vi "AlliGator Read HDF5 FLI Image Information.vi"(8 "error in (no error)":errorcluster, 11 "ref in":T3 format="%.0x") -> (0 "error out":errorcluster, 1 "Image Information":string, 2 "Image Binning Options":T1={"Use Image Binning"=FALSE, "X Bin"=1, "Y Bin"=1} {"Y Bin" min=1; "X Bin" min=1}, 3 "Image ROI Information":T2)   [LabVIEW 2021, in "AlliGator HDF5.lvlib"]
doc: "Reads HDF5 FLI dataset image information."
uses:
  AlliGator HDF5.lvlib
  <vilib>/addons/h5labview2/base/hid_t.ctl
  SwissSPAD/SwissSPAD Live_Image ROI Information.ctl
  AlliGator Image Binning Options.ctl
  <vilib>/addons/h5labview2/base/lib_path.vi
  <vilib>/addons/h5labview2/base/H5Equery.vi
  <vilib>/addons/h5labview2/dataset/H5Dread.llb/H5Dread.xnode
  SwissSPAD/SwissSPAD Live.lvlib
  AlliGator Source Image.lvlib
  <vilib>/addons/h5labview2/group/H5G.lvlib
  Variant/Variant.lvlib
panel:
  # "see the AlliGator License on the block diagram (Ctrl+E or Window:Show Block Diagram)"
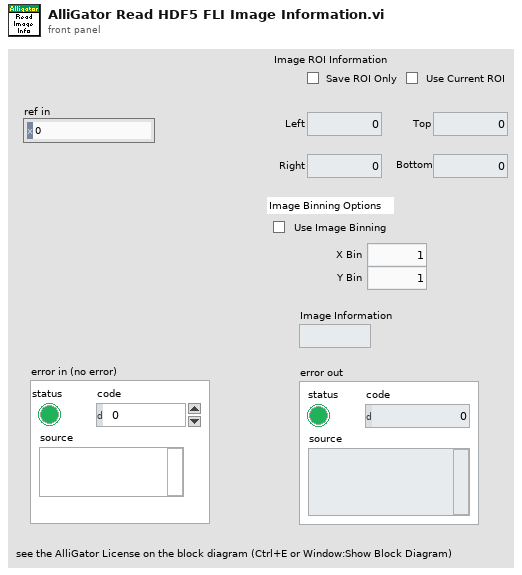
[diagram p1: front panel]
types:
  T1 = typedef "AlliGator Source Image.lvlib/AlliGator Image Binning Options.ctl" = cluster{"Use Image Binning":bool, "X Bin":i32, "Y Bin":i32}
  T2 = typedef "SwissSPAD Live.lvlib/SwissSPAD Live_Image ROI Information.ctl" = cluster{"Save ROI Only":bool, "Left":u16, "Top":u16, "Right":u16, "Bottom":u16, "Use Current ROI":bool}
  T3 = typedef "hid_t.ctl" = i64
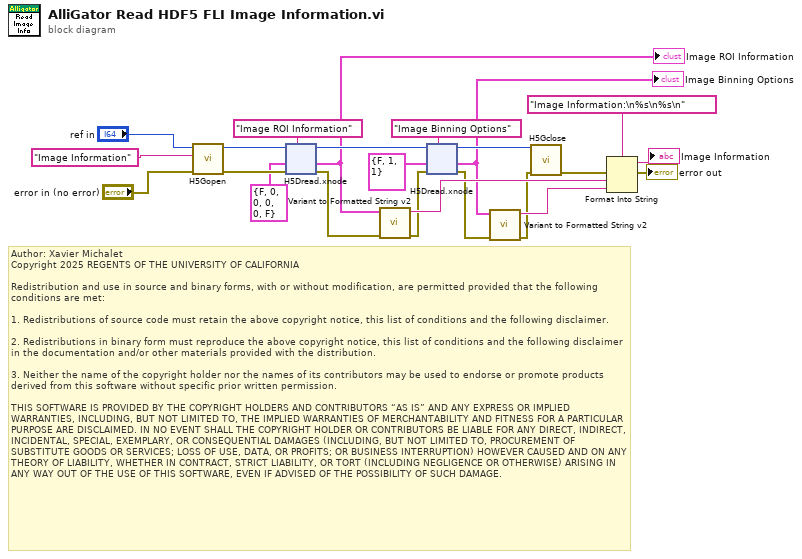
[diagram p0: block diagram]
diagram:
  # "Author: Xavier Michalet\nCopyright 2025 REGENTS OF THE UNIVERSITY OF CALIFORNIA\n\nRedistribution and use in source and binary forms, with or without modification, are permitted provided that the following conditions are met:\n\n1. Redistributions of source code must retain the above copyright notice, this list of conditions and the following disclaimer.\n\n2. Redistributions in binary form must reproduce the above copyright notice, this list of conditions and the following disclaimer in the documentation and/or other materials provided with the distribution.\n\n3. Neither the name of the copyright holder nor the names of its contributors may be used to endorse or promote products derived from this software without specific prior written permission.\n\nTHIS SOFTWARE IS PROVIDED BY THE COPYRIGHT HOLDERS AND CONTRIBUTORS “AS IS” AND ANY EXPRESS OR IMPLIED WARRANTIES, INCLUDING, BUT NOT LIMITED TO, THE IMPLIED WARRANTIES OF MERCHANTABILITY AND FITNESS FOR A PARTICULAR PURPOSE ARE DISCLAIMED. IN NO EVENT SHALL THE COPYRIGHT HOLDER OR CONTRIBUTORS BE LIABLE FOR ANY DIRECT, INDIRECT, INCIDENTAL, SPECIAL, EXEMPLARY, OR CONSEQUENTIAL DAMAGES (INCLUDING, BUT NOT LIMITED TO, PROCUREMENT OF SUBSTITUTE GOODS OR SERVICES; LOSS OF USE, DATA, OR PROFITS; OR BUSINESS INTERRUPTION) HOWEVER CAUSED AND ON ANY THEORY OF LIABILITY, WHETHER IN CONTRACT, STRICT LIABILITY, OR TORT (INCLUDING NEGLIGENCE OR OTHERWISE) ARISING IN ANY WAY OUT OF THE USE OF THIS SOFTWARE, EVEN IF ADVISED OF THE POSSIBILITY OF SUCH DAMAGE."
  n1 = call <vilib>:"H5Gopen.vi"("error in (no error)"="error in (no error)", "name"="Image Information" ("dataset name (this)"), "ref in"="ref in") -> ("error out"=w13:errorcluster, "group out"=w14:T3)  [unwired: 7 in]
  n2 = xnode "H5Dread.xnode"("dataset name (this)"="Image ROI Information" ("name"), "error in (no error)"=w13, "default"=T2 {"Save ROI Only"=FALSE, "Left"=0, "Top"=0, "Right"=0, "Bottom"=0, "Use Current ROI"=FALSE} ("Image Information"), "ref in"=w14) -> ("error out"=w7:errorcluster, "data"=w8:T2, "ref out"=w9:T3)  [unwired: 2 in, 1 out]
  "Image ROI Information" <- w8
  n3 = call "Variant to Formatted String v2.vi"("error in (no error)"=w7, "Anything"=w8) -> ("error out"=w10:errorcluster, "String"=w22:string)  [unwired: 8 in]
  n4 = xnode "H5Dread.xnode"("dataset name (this)"="Image Binning Options" ("name"), "error in (no error)"=w10, "default"=T1 {"Use Image Binning"=FALSE, "X Bin"=1, "Y Bin"=1} ("Image Binning Options"), "ref in"=w9) -> ("error out"=w17:errorcluster, "data"=w12:T1, "ref out"=w16:i64)  [unwired: 2 in, 1 out]
  "Image Binning Options" <- w12
  n5 = call "Variant to Formatted String v2.vi"("error in (no error)"=w17, "Anything"=w12) -> ("error out"=w18:errorcluster, "String"=w23:string)  [unwired: 8 in]
  n6 = call <vilib>:"H5Gclose.vi"("error in (no error)"=w18, "group in"=w16) -> ("error out"=w21:errorcluster)  [unwired: 9 in]
  n7 = Format Into String(format string="Image Information:\n%s\n%s\n", error in=w21, w22, w23) -> (resulting string=→"Image Information":string, error out=→"error out":errorcluster)  [unwired: 1 in]
